vi "WRO2018.vi"   [LabVIEW 2017]
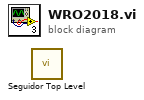
[diagram p0: block diagram]
diagram:
  n1 = call "Seguidor Top Level.vi"() -> ()  [unwired: 15 in, 1 out]
